vi "filter.test.AddOrder.and.OrderExecuted.vi"() -> ()   [LabVIEW 2020]
uses:
  fpga/common/orderbook.command.type.ctl
  fpga/common/orderbook.command.ctl
panel:
  out "GetState":u64[](array[numeric]) format="%.0x"
  in  "Expected.GetState":u64[](array[numeric])=[4702127773838221344, 176, 6076284164848492576, 177, 32, 20000, 48, 200] format="%.0x"
  out "error out":errorcluster
  out "Debug":u64[](array[numeric]) format="%.0x"
  out "Passed":bool
  out "OrderBook.Commands.out":T1[](array[typedef]) {"symbol" format="%.0x"; "orderId" format="%.0x"; "side" format="%.0x"}
  in  "OrderBook.Commands.in":T1[](array[typedef])=[{"type"=enum."AddOrder", "side"=66, "orderId "=48, "quantity"=20000, "symbol"=4702127773838221344, "price"=9050, "executed.qty"=0, "canceled.qty"=0, "remaining.qty"=0, "seconds"=0, "nanoseconds"=0, "Add"=FALSE, "Edit"=FALSE, "Remove"=FALSE}, {"type"=enum."ModifyOrder", "side"=66, "orderId "=48, "quantity"=200, "symbol"=0, "price"=9050, "executed.qty"=0, "canceled.qty"=0, "remaining.qty"=0, "seconds"=0, "nanoseconds"=0, "Add"=FALSE, "Edit"=FALSE, "Remove"=FALSE}, {"type"=enum."AddOrder", "side"=66, "orderId "=32, "quantity"=20000, "symbol"=6076284164848492576, "price"=9050, "executed.qty"=0, "canceled.qty"=0, "remaining.qty"=0, "seconds"=0, "nanoseconds"=0, "Add"=FALSE, "Edit"=FALSE, "Remove"=FALSE}] {"symbol" format="%.0x"; "orderId" format="%.0x"; "side" format="%.0x"}
  in  "Watch.List":string[](array[string])=["AAPL", "TSLA"]
  in  "Expected OrderBook.Commands":T1[](array[typedef])=[{"type"=enum."AddOrder", "side"=66, "orderId "=48, "quantity"=20000, "symbol"=4702127773838221344, "price"=9050, "executed.qty"=0, "canceled.qty"=0, "remaining.qty"=0, "seconds"=0, "nanoseconds"=0, "Add"=FALSE, "Edit"=FALSE, "Remove"=FALSE}, {"type"=enum."ModifyOrder", "side"=66, "orderId "=48, "quantity"=200, "symbol"=0, "price"=9050, "executed.qty"=0, "canceled.qty"=0, "remaining.qty"=0, "seconds"=0, "nanoseconds"=0, "Add"=FALSE, "Edit"=FALSE, "Remove"=FALSE}, {"type"=enum."AddOrder", "side"=66, "orderId "=32, "quantity"=20000, "symbol"=6076284164848492576, "price"=9050, "executed.qty"=0, "canceled.qty"=0, "remaining.qty"=0, "seconds"=0, "nanoseconds"=0, "Add"=FALSE, "Edit"=FALSE, "Remove"=FALSE}] {"symbol" format="%.0x"; "orderId" format="%.0x"; "side" format="%.0x"}
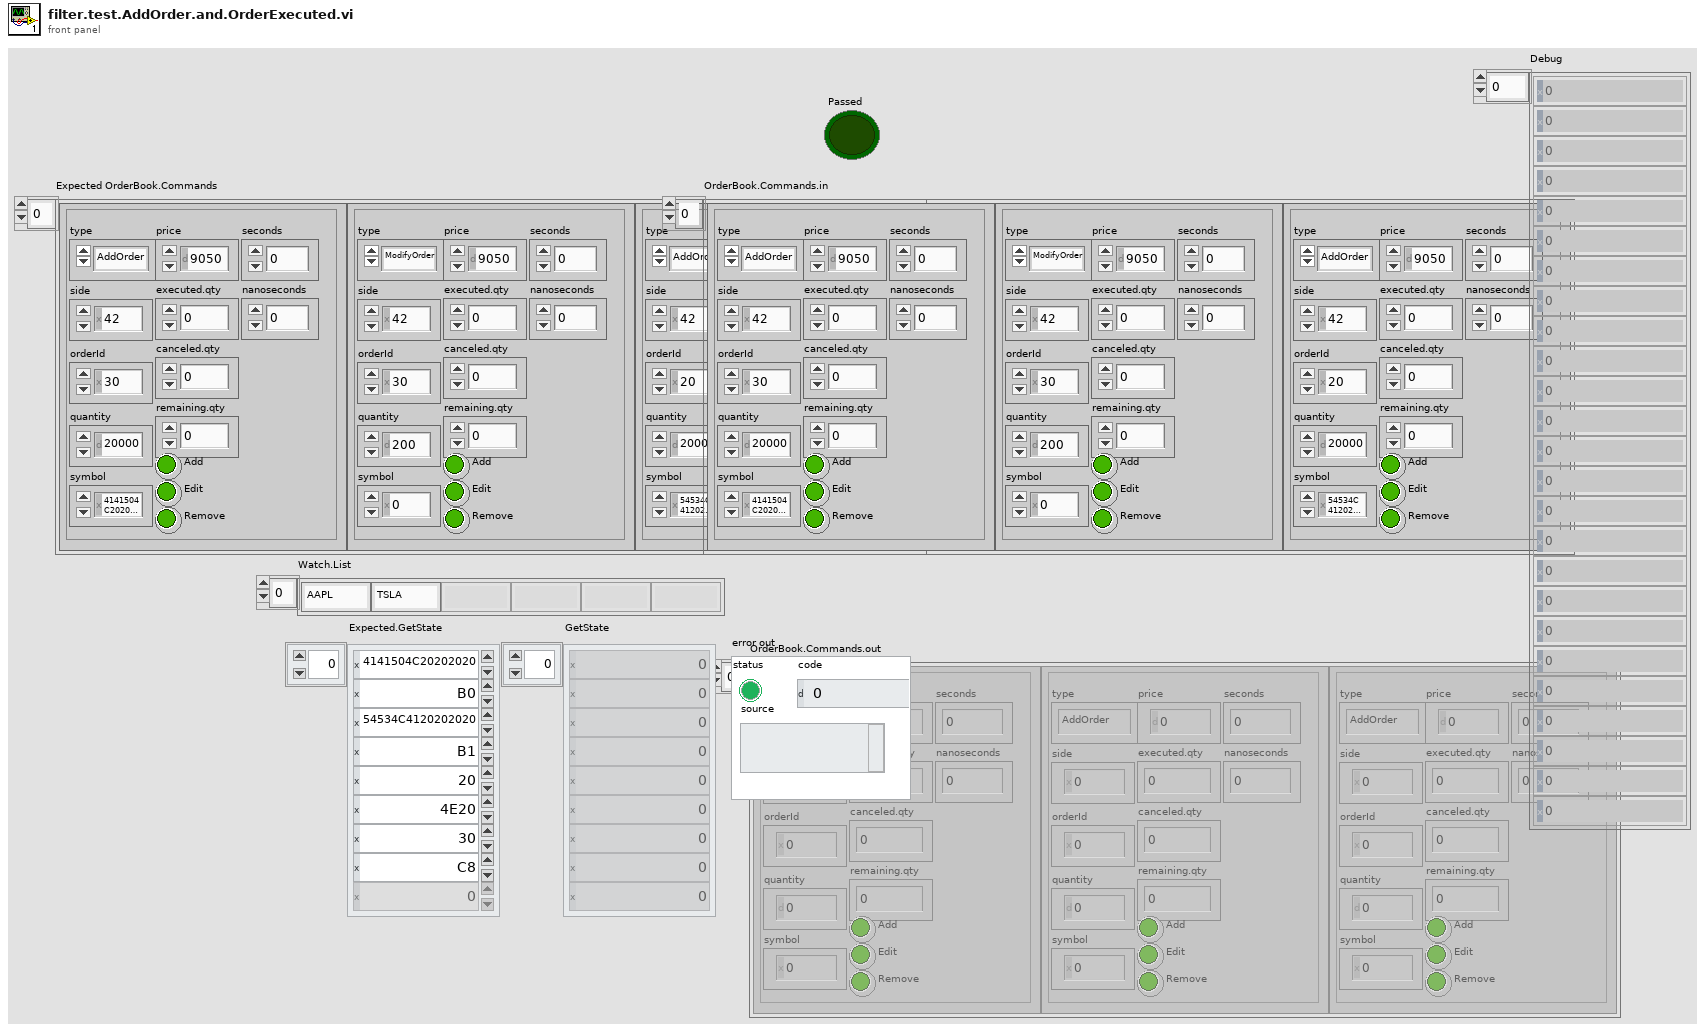
[diagram p1: front panel]
types:
  T1 = typedef "orderbook.command.ctl" = cluster{"type":T2, "side":u8, "orderId ":u64, "quantity":u32, "symbol":u64, "price":u64, "executed.qty":u32, "canceled.qty":u32, "remaining.qty":u32, "seconds":u64, "nanoseconds":u64, "Add":bool, "Edit":bool, "Remove":bool}
  T2 = typedef "orderbook.command.type.ctl" = enum8{"Time", "AddOrder", "OrderExecuted", "OrderExecutedAtPrice", "ReduceSize", "ModifyOrder", "DeleteOrder", "Get.Everything", "Get.All.Orders", "Get.Top"}
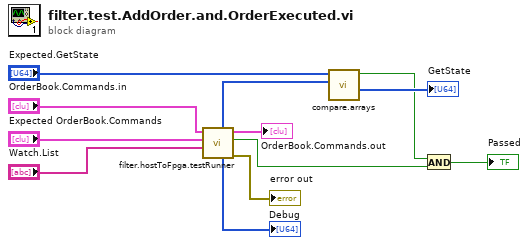
[diagram p0: block diagram]
diagram:
  n1 = call "filter.hostToFpga.testRunner.vi"("Watch.List"="Watch.List", "Expected OrderBook.Command[]"="Expected OrderBook.Commands", "OrderBook.Commands.in"="OrderBook.Commands.in") -> ("error out"=→"error out":errorcluster, "Passed"=w6:bool, "OrderBook.Commands.out"=→"OrderBook.Commands.out":T1[], "Debug"=→"Debug":u64[], "GetState"=w1:u64[])  [unwired: 2 in, 2 out]
  n2 = call "compare.arrays.vi"("Actual"=w1, "Expected"="Expected.GetState") -> ("Actual.Out"=→"GetState":u64[], "Full.Match"=w3:bool)  [unwired: 7 in, 1 out]
  n3 = And(x=w3, y=w6) -> (x .and. y?=→"Passed":bool)
